vi "Find Other Xnode Instances in Same VI.vi"(4 "Error In":errorcluster, 7 "XRef":T1) -> (0 "Error Out":errorcluster, 2 "Other XNode Instances":T1[](array[typedef]))   [LabVIEW 2025, in "XNode Support.lvlib"]
doc: "Finds all instances of \"Decoration Reference.xnode\" in same VI"
uses:
  XNode Support.lvlib
  <vilib>/XNodeSupport/XNodeXNodeRef.ctl
  <vilib>/Utility/traverseref.llb/TRef TravTarget.ctl
  <vilib>/Utility/traverseref.llb/VI Scripting - Traverse.lvlib
  <vilib>/XNodeSupport/NI_XNodeSupport.lvlib
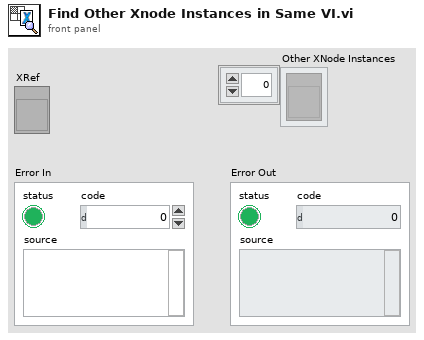
[diagram p1: front panel]
types:
  T1 = typedef "NI_XNodeSupport.lvlib/XNodeXNodeRef.ctl" = refnum<vi>
  T2 = typedef "TRef TravTarget.ctl" = enum16{"FP", "BD", "Other"}
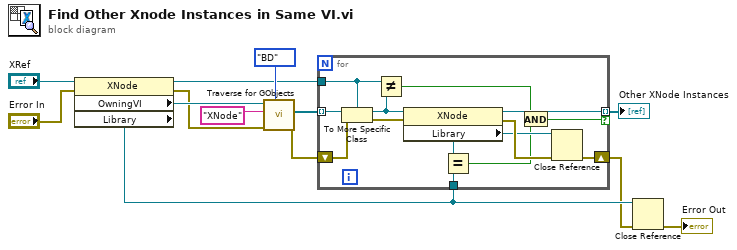
[diagram p0: block diagram]
diagram:
  n1 = property class="XNode"(reference="XRef", error in="Error In") -> (reference out=w6:T1, error out=w11:errorcluster, "OwningVI"=w12:refnum<vi>, "Library"=w4:refnum<vi>)
  n2 = call <vilib>:"Traverse for GObjects.vi"("Traverse Target"=TRef_TravTarget."BD", "error in (no error)"=w11, "Class Name"="XNode", "VI Refnum"=w12) -> ("error out"=w7:errorcluster, "References"=w8:refnum<vi>[])  [unwired: 4 in, 2 out]
  n3 = for {
    tunnel: w8 -> [w26] mode=indexing
    tunnel: w6 -> [w18]
    tunnel: w4 -> [w23]
    tunnel: [w22] -> w1 mode=indexing if=w14
    shift-right: [w19] -> w3
    shift-left: w7 -> [w25]
    n4 = To More Specific Class(target class=w18, reference=w26, error in=w25) -> (specific class reference=w17:T1, error out=w24:errorcluster)
    n5 = Not Equal?(x=w18, y=w17) -> (x != y?=w16:bool)
    n6 = property class="XNode"(reference=w17, error in=w24) -> (reference out=w22:T1, error out=w21:errorcluster, "Library"=w20:refnum<vi>)
    n7 = Equal?(x=w20, y=w23) -> (x = y?=w15:bool)
    n8 = And(x=w16, y=w15) -> (x .and. y?=w14:bool)
    n9 = Close Reference(reference=w20, error in (no error)=w21) -> (error out=w19:errorcluster)
  }
  "Other XNode Instances" <- w1
  n10 = Close Reference(reference=w4, error in (no error)=w3) -> (error out=→"Error Out":errorcluster)
